vi "Apply Rove.vi"(8 "error in (no error)":errorcluster, 11 "TTLControl in":refnum<class "TTLController.lvclass">) -> (0 "error out":errorcluster, 1 "DisplayString":string[](array[string]), 2 "FileString":string[](array[string]), 3 "TTLControl out":refnum<class "TTLController.lvclass">)   [LabVIEW 2020, in "TTLController.lvclass"]
uses:
  TTLController.lvclass
  TTLController.lvclass/TTLController.ctl
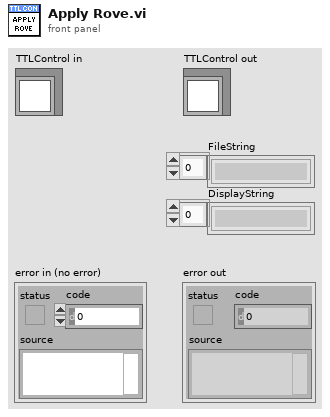
[diagram p1: front panel]
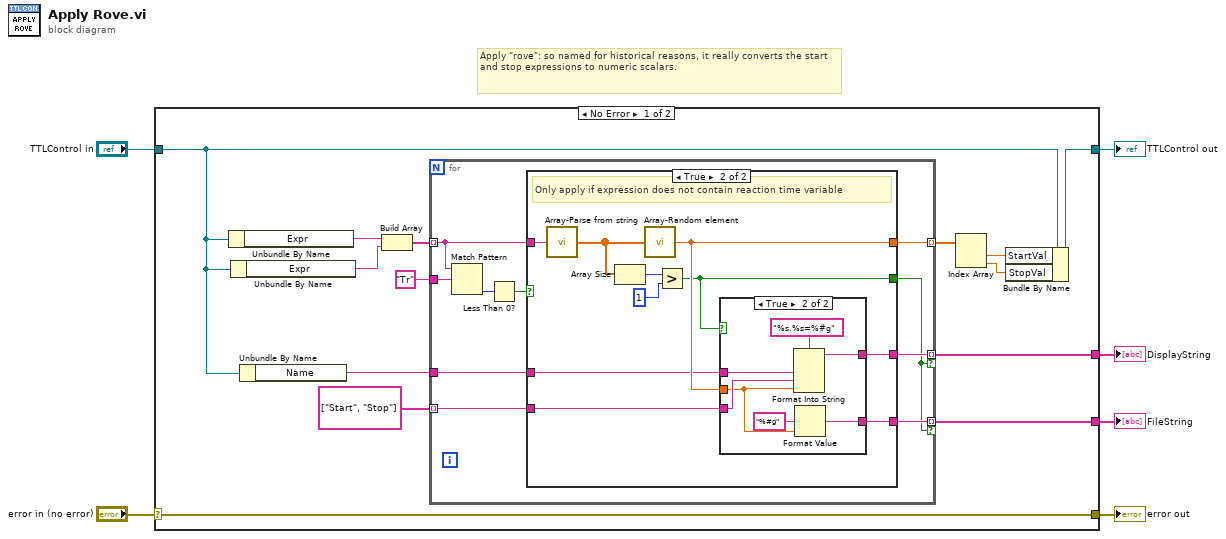
[diagram p0: block diagram]
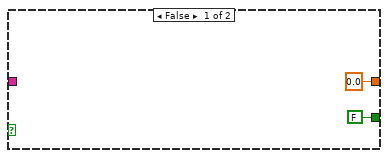
[diagram p2: hidden frame]
diagram:
  # "Apply \"rove\": so named for historical reasons, it really converts the start and stop expressions to numeric scalars."
  n1 = case shown="No Error" "error in (no error)" {
    selector: "error in (no error)" -> [w20 w51]
    tunnel: [w20 w51] -> w5
    tunnel: [w18 w50] -> w3
    tunnel: "TTLControl in" -> [w17 w50]
    tunnel: [w9 _] -> w2
    tunnel: [w8 _] -> w1
    frame No Error {
      n2 = Unbundle By Name(w17) -> ("Expr"=w19:string)
      n3 = Unbundle By Name(w17) -> ("Expr"=w14:string)
      n4 = Unbundle By Name(w17) -> ("Name"=w16:string)
      n5 = Build Array(w19, w14) -> (w15:string[])
      n6 = for {
        tunnel: w15 -> [w24] mode=indexing
        tunnel: [w30] -> w12 mode=indexing
        tunnel: w16 -> [w29]
        tunnel: string[] ["Start", "Stop"] -> [w28] mode=indexing
        tunnel: [w27] -> w9 mode=indexing if=w25
        tunnel: [w26] -> w8 mode=indexing if=w25
        tunnel: "Tr" -> [w23]
        n7 = Match Pattern(string=w24, regular expression=w23) -> (offset past match=w22:i32)  [unwired: 1 in, 3 out]
        n8 = Less Than 0?(x=w22) -> (x < 0?=w21:bool)
        n9 = case shown="True" w21 {
          tunnel: [0.0 ("Element") w40] -> w30
          tunnel: w29 -> [_ w39]
          tunnel: w28 -> [_ w38]
          tunnel: [_ w37] -> w27
          tunnel: [_ w36] -> w26
          tunnel: [FALSE w35] -> w25
          tunnel: w24 -> [_ w33]
          frame False {
          }
          frame True {
            # "Only apply if expression does not contain reaction time variable"
            n10 = call "Array-Parse from string.vi"("String"=w33) -> ("Array"=w42:dbl[])  [unwired: 13 in, 1 out]
            n11 = Array Size(array=w42) -> (size(s)=w41:i32)
            n12 = call "Array-Random element.vi"("Array"=w42) -> ("Element"=w40:dbl)  [unwired: 1 in, 1 out]
            n13 = Greater?(x=w41, y=1) -> (0:w35:bool)
            n14 = case shown="True" w35 {
              tunnel: w40 -> [_ w46]
              tunnel: w39 -> [_ w48]
              tunnel: w38 -> [_ w47]
              tunnel: [_ w44] -> w37
              tunnel: [_ w43] -> w36
              frame False {
              }
              frame True {
                n15 = Format Into String(format string="%s.%s=%#g", w48, w47, w46) -> (resulting string=w44:string)  [unwired: 2 in, 1 out]
                n16 = Format Value(format string="%#g", value (0)=w46) -> (output string=w43:string)  [unwired: 1 in]
              }
            }
          }
        }
      }
      n17 = Index Array(array=w12) -> (element #1=w11:dbl, element #2=w10:dbl)  [unwired: 2 in]
      n18 = Bundle By Name(cluster=w17, "StartVal"=w11, "StopVal"=w10) -> (w18:refnum<class "TTLController.lvclass">)
    }
    frame Error {
    }
  }
  "error out" <- w5
  "TTLControl out" <- w3
  "FileString" <- w1
  "DisplayString" <- w2
